vi "Write-Read Mux Message.vi"(8 "error in":errorcluster, 9 "Channel":string, 10 "ASIC":dbl, 11 "VISA in":refnum<visa-resource-name>) -> (0 "error out":errorcluster, 2 "read buffer":string)   [LabVIEW 2019]
uses:
  <vilib>/Instr/_visa.llb/VISA Configure Serial Port (Instr).vi
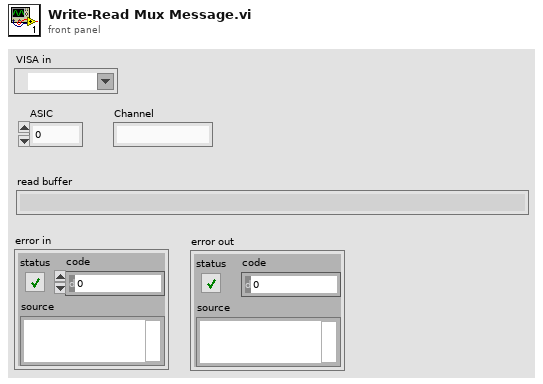
[diagram p1: front panel]
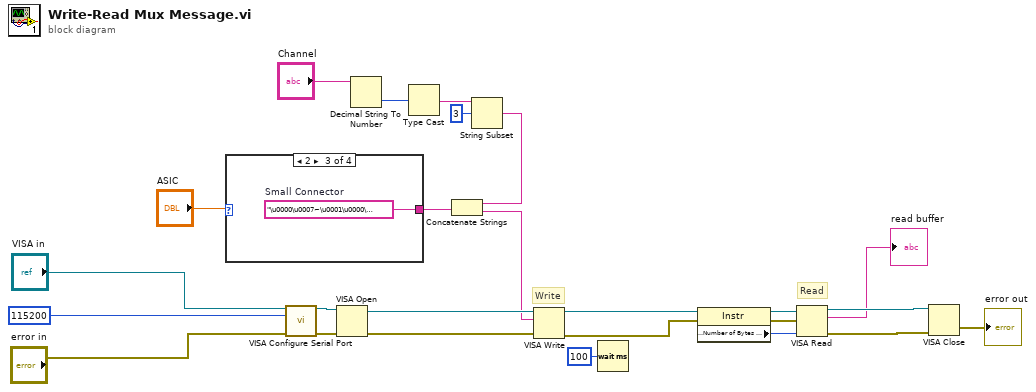
[diagram p0: block diagram]
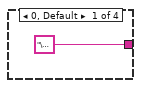
[diagram p2: hidden frame]
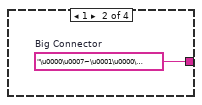
[diagram p3: hidden frame]
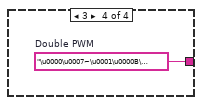
[diagram p4: hidden frame]
diagram:
  # "Write"
  # "Read"
  n1 = case shown="2" "ASIC" {
    tunnel: ["\u0000" w27 w28 w29] -> w4
    frame 0, Default {
    }
    frame 1 {
      w27 = "\u0000\u0007~\u0001\u0000\u0010„‡+"  # Big Connector
    }
    frame 2 {
      w28 = "\u0000\u0007~\u0001\u0000\u0010HŸë"  # Small Connector
    }
    frame 3 {
      w29 = "\u0000\u0007~\u0001\u0000B\u0018­Ã"  # Double PWM
    }
  }
  n2 = call-poly "VISA Configure Serial Port"("VISA resource name"="VISA in", "baud rate (9600)"=u32 115200, "error in (no error)"="error in") -> ("VISA resource name out"=w23:refnum<visa-resource-name>, "error out"=w24:errorcluster)  [unwired: 11 in]
  n3 = VISA Open(error in (no error)=w24, VISA resource name=w23) -> (VISA resource name=w17:refnum<visa-resource-name>, error out=w18:errorcluster)  [unwired: 3 in]
  n4 = Decimal String To Number(string="Channel") -> (number=w19:i32)  [unwired: 2 in, 1 out]
  n5 = Type Cast(x=w19) -> (*(type *) &x=w20:string)  [unwired: 1 in]
  n6 = String Subset(string=w20, offset (0)=3) -> (substring=w22:string)  [unwired: 1 in]
  n7 = Concatenate Strings(w22, w4) -> (w3:string)
  n8 = VISA Write(VISA resource name=w17, write buffer=w3, error in (no error)=w18) -> (VISA resource name out=w12:refnum<visa-resource-name>, error out=w13:errorcluster)  [unwired: 1 out]
  n9 = Wait (ms)(milliseconds to wait=u32 100) -> ()  [unwired: 1 out]
  n10 = property class="Instr"(reference=w12, error in=w13) -> (reference out=w14:refnum<visa-resource-name>, error out=w15:errorcluster, "Serial Settings:Number of Bytes at Serial Port"=w16:u32)
  n11 = VISA Read(VISA resource name=w14, byte count=w16, error in (no error)=w15) -> (VISA resource name out=w10:refnum<visa-resource-name>, read buffer=→"read buffer":string, error out=w11:errorcluster)  [unwired: 1 out]
  n12 = VISA Close(VISA resource name=w10, error in (no error)=w11) -> (error out=→"error out":errorcluster)
